vi "configureTiming.vi"(2 "error in (no error)":errorcluster, 3 "Timing":T1, 4 "AnalogOutput in":refnum<class "AnalogOutput.lvclass">) -> (0 "error out":errorcluster, 1 "AnalogOutput out":refnum<class "AnalogOutput.lvclass">)   [LabVIEW 2009, in "Hardware.lvlib" / "Channels.lvlib" / "AnalogOutput.lvclass"]
doc: "Abstract Method.\n\nUse this method after configureForVoltageOutput.vi, to set the timing and triggering information which the analog output requires. This method store this information in the classes data, and then calls setTiming.vi which is implemented by child classes to interact with the specific hardware device. \n\nThe Cluster passed in here includes:\n1) Clock source (String, example \"/DAQ/PXI_Clk10\")\n2) Clock rate (Double, example \"10E+6\" 10MHz)\n3) Start trigger line (String, example \"/Ao32/PXI_Trig0\")\n4) Sample Rate (Double, example \"1E+6\" 1MS/s)\n5) Number of Samples (Double, example \"10E+6\" = 10 seconds of data)"
uses:
  AnalogOutput.lvclass
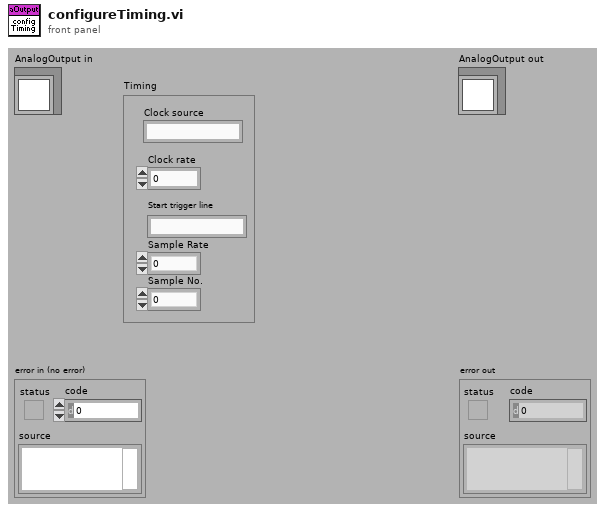
[diagram p1: front panel]
types:
  T1 = cluster{"Clock source":string, "Clock rate":dbl, "Start trigger line":string, "Sample Rate":dbl, "Sample No.":dbl}
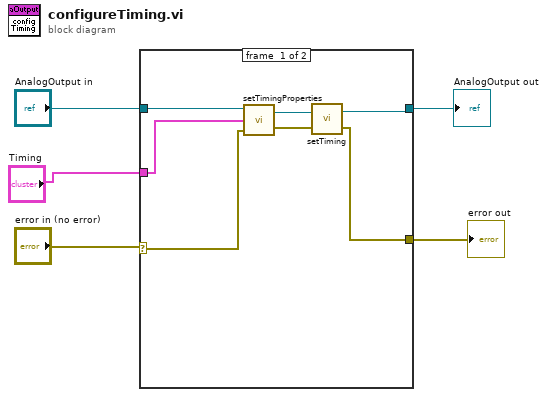
[diagram p0: block diagram]
diagram:
  n1 = case shown="No Error" "error in (no error)" {
    selector: "error in (no error)" -> [w11 w14]
    tunnel: [w6 w14] -> w4
    tunnel: [w7 w13] -> w2
    tunnel: "AnalogOutput in" -> [w12 w13]
    tunnel: "Timing" -> [w10 _]
    frame #0 {
      n2 = call "setTimingProperties.vi"("error in (no error)"=w11, "Timing"=w10, "AnalogOutput.lvclass in"=w12) -> ("error out"=w8:errorcluster, "AnalogOutput.lvclass out"=w9:refnum<class "AnalogOutput.lvclass">)
      n3 = call-dynamic "setTiming.vi"("error in (no error)"=w8, "AnalogOutput in"=w9) -> ("error out"=w6:errorcluster, "AnalogOutput out"=w7:refnum<class "AnalogOutput.lvclass">)
    }
    frame #1 {
    }
  }
  "error out" <- w4
  "AnalogOutput out" <- w2
